vi "告警触发机制 (子VI).vi"(9 "声光告警启用":bool, 10 "状态输出":bool, 11 "Digital输入":refnum<vi>) -> (2 "声光告警":bool, 3 "触发告警":bool)   [LabVIEW 2016, in "环境动力监测库.lvlib"]
uses:
  <vilib>/ptbypt/NI_PtbyPt.lvlib
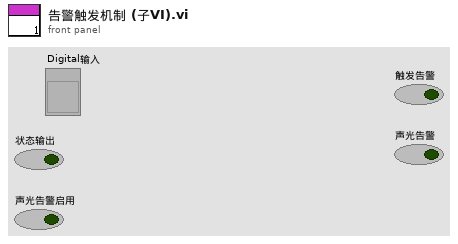
[diagram p1: front panel]
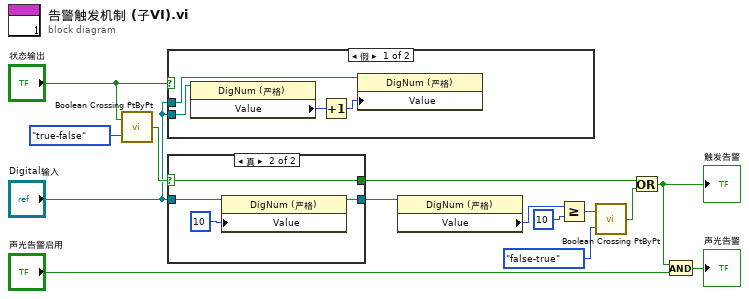
[diagram p0: block diagram]
diagram:
  n1 = call <vilib>:"Boolean Crossing PtByPt.vi"("direction"=enum16{"either", "false-true", "true-false"}."true-false", "input"="状态输出") -> ("crossing"=w4:bool)  [unwired: 1 in]
  n2 = case shown="假" "状态输出" {
    tunnel: "Digital输入" -> [w16 _]
    tunnel: "Digital输入" -> [w15 _]
    frame False {
      n3 = property class="DigNum (严格)"(reference=w16) -> ("Value"=w17:u32)  [unwired: 1 in, 2 out]
      n4 = Increment(x=w17) -> (x+1=w18:u32)
      n5 = property class="DigNum (严格)"(reference=w15, "Value"=w18) -> ()  [unwired: 1 in, 2 out]
    }
    frame True {
    }
  }
  n6 = case shown="真" w4 {
    selector: w4 -> [w19 w21]
    tunnel: "Digital输入" -> [w20 w24]
    tunnel: [w20 w22] -> w3
    tunnel: [w19 w21] -> w2
    frame False {
    }
    frame True {
      n7 = property class="DigNum (严格)"(reference=w24, "Value"=u32 10 ("值")) -> (reference out=w22:refnum<vi>)  [unwired: 1 in, 1 out]
    }
  }
  n8 = property class="DigNum (严格)"(reference=w3) -> ("Value"=w7:u32)  [unwired: 1 in, 2 out]
  n9 = Greater Or Equal?(x=w7, y=u32 10) -> (x >= y?=w12:bool)
  n10 = call <vilib>:"Boolean Crossing PtByPt.vi"("direction"=enum16{"either", "false-true", "true-false"}."false-true", "input"=w12) -> ("crossing"=w14:bool)  [unwired: 1 in]
  n11 = Or(x=w2, y=w14) -> (x .or. y?=w10:bool)
  "触发告警" <- w10
  n12 = And(x=w10, y="声光告警启用") -> (x .and. y?=→"声光告警":bool)
